vi "#SPI_TOF_LIDAR_cz_test.vi"() -> ()   [LabVIEW 2020]
uses:
  <vilib>/Analysis/baseanly.llb/Mean (DBL).vi
  handle_ALP_error.vi
  <vilib>/Utility/error.llb/Error Cluster From Error Code.vi
  <vilib>/Analysis/NI_AALBase.lvlib
  <vilib>/gmath/NI_Gmath.lvlib
panel:
  out "Trigger Delay (samples)":u32
  out "Rapid Block Acquisition Settings":T1={"preTriggerSamples"=0, "postTriggerSamples"=1000, "timebase"=2, "Four Channel Device"=FALSE, "Oversample"=1, "Number of Captures"=1}
  in  "Tab Control 2":T2(tab)
  out "Resolution":i32=32 min=16 max=128 step=16
  in  "Max Resolution":enum16{"128", "64", "32", "16"}(ring)=enum."32"
  in  "Pulses/Pattern":i32=4
  in  "Trigger Settings":T3={"Trigger Enabled"=TRUE, "Trigger Source"=enum."Channel C", "Trigger Threshold"=10, "Trigger Direction"=2, "Trigger Delay (samples)"=40, "Auto Trigger Time (ms)"=1000} {"Trigger Direction" items=["Rising"=2, "Falling"=3]}
  out "Captures":u32=10240
  in  "Post Trig. Samples":u32=30
  out "Patterns Loaded":dbl(slide)=2048.0 scale=0.0..2048.0
  in  "Initialised?":bool
  in  "y":dbl=0.9
  out "picture time s":dbl=0.0005142857142857143 format="%#.3p"
  in  "Pre Trigger Samples":u32
  in  "Patterns":enum16{"Hadamard", "Random", "Democratised"}(ring)
  in  "Smooth (pixels)":dbl=0.4 format="%#_13g"
  in  "ntimes":i32=4
  in  "Thresholded":bool
  in  "First":bool
  in  "upsample factor":i32=1
  in  "Depth Smooth":dbl=1.0 format="%#_13g"
  in  "depth threshold":dbl=1.0000000000000009
  in  "reflectivity threshold":dbl=0.35 format="%#_13g"
  in  "max reflectivity":dbl=1.0
  in  "index (row)":i32
  in  "Additional Data":dbl=1.25 format="%#_13g"
  out "# elements 2":i32
  out "Total Rate (Hz)":dbl=45.45454545454545 format="%.2g"
  out "# elements 3":i32
  out "2D Rate (Hz)":dbl=inf format="%.2g"
  out "3D Rate (Hz)":dbl=inf format="%.2g"
  out "Update Rate (Hz)":dbl=45.45454545454545 format="%.2g"
  in  "Tab Control":T4(tab)=enum."Temporal Signals"
  out "?":dbl[](graph)
  out "?":dbl[](graph)
  out "pattern temporal signal":cluster{dbl[], dbl[]}(graph)
  out "?":dbl[](graph)
  out "Depth Map":dbl[][](graph)
  out "Reconstruction":dbl[][](graph)
  out "Hadamards":bool[][](array[boolean])
  in  "Channel A Settings":T5={"Enabled"=TRUE, "Coupling"=2, "Range"=3, "Analogue Offset"=0.0, "Bandwidth"=0} {"Bandwidth" items=["Full", "20 MHz"]; "Range" items=["10 mV", "20 mV", "50 mV", "100 mV", "200 mV", "500 mV", "1 V", "2 V", "5 V", "10 V", "20 V", "50 V ", "100 V"]; "Coupling" items=["AC", "DC 1 MOhm", "DC 50 Ohm"]}
  out "total patterns":i32=2048
  in  "Stop":bool=TRUE
  # "3000"
  # "maxADC=32512"
  # "400ps per delay point"
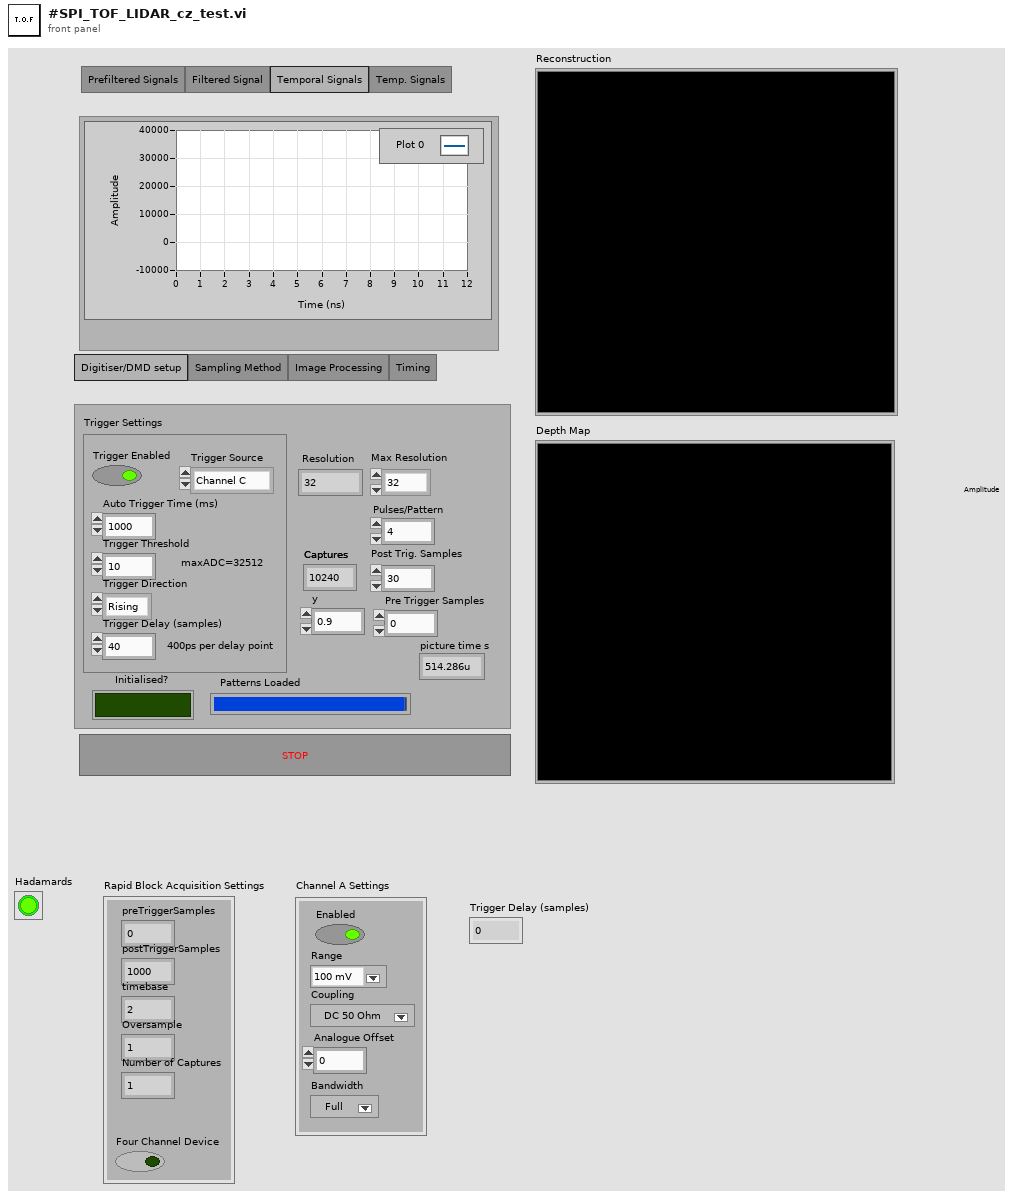
[diagram p1: front panel]
types:
  T1 = cluster{"preTriggerSamples":u32, "postTriggerSamples":u32, "timebase":u32, "Four Channel Device":bool, "Oversample":i16, "Number of Captures":u32}
  T2 = enum32{"Digitiser/DMD setup", "Sampling Method", "Image Processing", "Timing"}
  T3 = cluster{"Trigger Enabled":bool, "Trigger Source":enum32{"Channel A", "Channel B", "Channel C", "Channel D", "External", "Aux."}, "Trigger Threshold":i16, "Trigger Direction":u16, "Trigger Delay (samples)":u32, "Auto Trigger Time (ms)":i16}
  T4 = enum32{"Prefiltered Signals", "Filtered Signal", "Temporal Signals", "Temp. Signals"}
  T5 = cluster{"Enabled":bool, "Coupling":u32, "Range":u32, "Analogue Offset":sgl, "Bandwidth":u32}
  T6 = cluster{dbl[][], "All Patterns out":bool[][], "LUT":i32[]}
  T7 = typedef "imagedata.ctl" = cluster{"image type":i32, "image depth":i32, "image":u8[], "mask":u8[], "colors":u32[], "Rectangle":cluster{"left":i16, "top":i16, "right":i16, "bottom":i16}}
  T8 = cluster{"Pre Trigger Samples":u32, "Post Trig. Samples":u32, "timebase":u32, "Four Channel Device":bool, "Oversample":i16, u32}
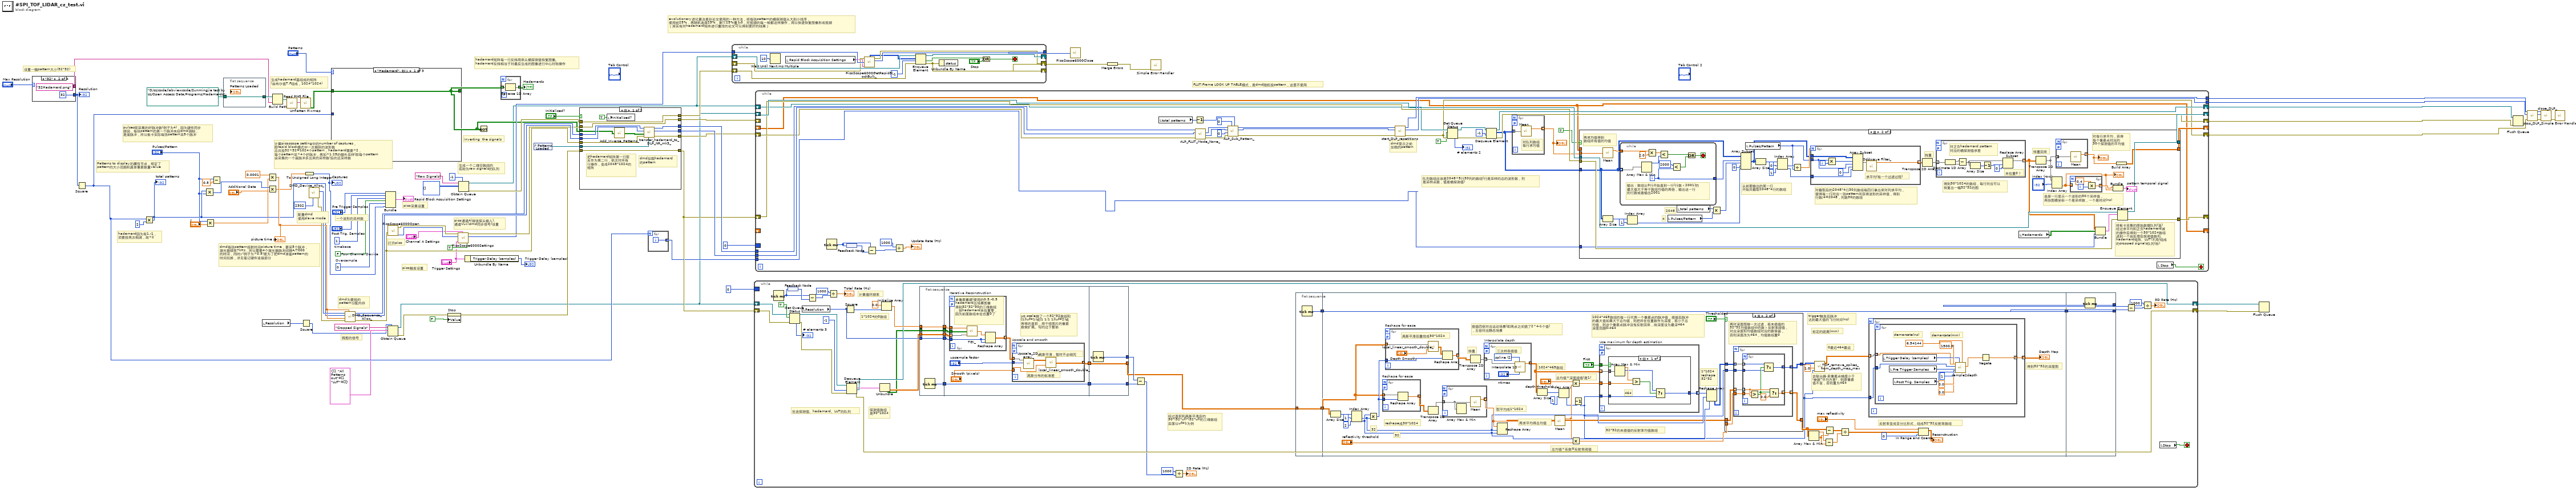
[diagram p0: block diagram]
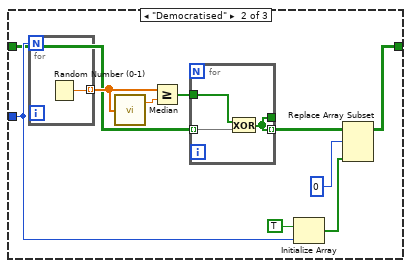
[diagram p2: hidden frame]
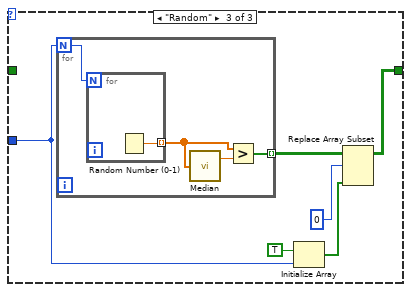
[diagram p3: hidden frame]
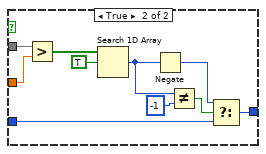
[diagram p5: hidden frame]
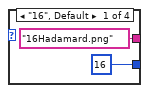
[diagram p8: hidden frame]
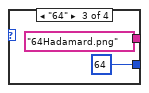
[diagram p9: hidden frame]
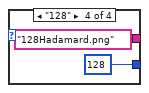
[diagram p10: hidden frame]
diagram:
  w10 = FALSE  # Four Channel Device
  w11 = u32 1  # timebase
  w8 = i16 0  # Oversample
  # "hadamard矩阵每一行反转用来从桶探测值恢复图像。\nhadamard反转相当于对最后生成的图像进行中心对称操作"
  # "pulses即采集的好脉冲数(例子为4)，因为硬件同步\n原因，每张pattern的第一个脉冲未经dmd调制，\n是废脉冲，所以板卡实际每张pattern采5个脉冲"
  # "裁剪的信号"
  # "evolutionary进化算法是孙论文使用的一种方法，将每张pattern的桶探测值从大到小排序，\n使用前25%，再随机选择25%，剩下25%置为0，对视频的每一帧都这样操作，用以快速恢复图像形成视频\n（其实有对hadamard矩阵进行重排的论文可以得到更好的结果）"
  # "生成一个二维空数组的\n名称为raw signals的队列"
  # "FLUT:Frame LOOK UP TABLE模式，是dmd随机投pattern，这里不使用"
  # "pico采集设置"
  # "pico通道A(接收探头输入).\n通道Vux(dmd同步信号)设置"
  # "pico触发设置"
  # "打开pico"
  # "配置dmd\n使用slave mode"
  # "dmd为要投的\npattern分配内存"
  # "dmd每张pattern投射时间picture time，要采5个脉冲，\n激光器频率7kHz，所以需要4个激光器脉冲间隔4/7000\n的时间，同时y(例子为×0.9)是为了把dmd准备pattern的\n时间扣掉，详见笔记硬件连接部分"
  # "一个波形的采样数"
  # "计算picoscope setting中的number of captures，\n即rapid block模式中一次捕获的波形数\n总共投32×32=1024个pattern，hadamard需要×2，\n每个pattern采×4个好脉冲，再加×1.25的额外采样(即每个pattern\n会采集的一个废脉冲多出来的采样数)后的总采样数"
  # "hadamard因为有1.-1，\n须要投两次相减，故×2"
  # "Patterns to display的属性节点，规定了\npattern的大小范围和具体像素数量value"
  # "生成hadamard基组成的矩阵\n(由布尔值T.F组成，1024*1024)"
  # "设置一幅pattern大小(32*32)"
  # "inverting  the signals"
  n1 = case shown="\"32\"" "Max Resolution" {
    tunnel: [16 32 64 128] -> w36
    tunnel: ["16Hadamard.png" ("string") "32Hadamard.png" ("string") "64Hadamard.png" ("string") "128Hadamard.png" ("string")] -> w24
    frame "16", Default {
    }
    frame "32" {
    }
    frame "64" {
    }
    frame "128" {
    }
  }
  "Resolution" <- w36
  n2 = Square(x=w36) -> (x^2=w34:i32)
  n3 = Multiply(x=w34, y=2) -> (x*y=w35:i32)
  "total patterns" <- w35
  n4 = Multiply(x=w35, y="Pulses/Pattern") -> (x*y=w54:i32)
  n5 = Multiply(x="Pulses/Pattern", y="y") -> (x*y=w20:dbl)
  n6 = Subtract(x="Pulses/Pattern", y=0.5) -> ()  [unwired: 1 out]
  n7 = flat-sequence {
    tunnel: path "D:/cz/code/labviewcode/Sunmingjie test by cz/Open Access Data/Programs/Hadamards" ("Folder to Store Files 2") -> [w91]
    tunnel: [w91] -> w25
    frame #0 {
    }
  }
  n8 = local read "Resolution"() -> (w52:i32)
  n9 = Multiply(x=0.0001, y=w20) -> (x*y=w76:dbl)
  "picture time s" <- w76
  n10 = Multiply(x=w54, y="Additional Data") -> (x*y=w60:dbl)
  n11 = Build Path(base path=w25, name or relative path=w24) -> (appended path=w23:path)
  n12 = call <vilib>:"Read PNG File.vi"("path to PNG file"=w23) -> ("image data"=w27:T7)  [unwired: 8 in, 2 out]
  n13 = call <vilib>:"Unflatten Pixmap.vi"("image data"=w27) -> ("1-bit pixmap"=w26:bool[][])  [unwired: 4 in, 6 out]
  n14 = Square(x=w52) -> (x^2=w16:i32)
  n15 = To Unsigned Long Integer(number=w60) -> (unsigned 32bit integer=w7:u32)
  "Captures" <- w7
  n16 = call "DMD_Device_Alloc_.vi"("Master/Slave Mode"=2302) -> ("error out"=w81:errorcluster, "DeviceIdPtr"=w82:u32)  [unwired: 8 in, 1 out]
  n17 = case shown="\"Hadamard\", 默认" "Patterns" {
    tunnel: w34 -> [_ w102 w108]
    tunnel: [w92 w98 w107] -> w18
    tunnel: w26 -> [w92 w96 _]
    frame "Hadamard", Default {
    }
    frame "Democratised" {
      n18 = for {
        N: w102 -> [_]
        tunnel: [w106] -> w97 mode=indexing
        n19 = Random Number (0-1)() -> (number: 0 to 1=w106:dbl)
      }
      n20 = call <vilib>:"Median.vi"("X"=w97) -> ("median"=w94:dbl)  [unwired: 1 out]
      n21 = Greater Or Equal?(x=w97, y=w94) -> (x >= y?=w93:bool[])
      n22 = for {
        tunnel: w93 -> [w105]
        tunnel: w96 -> [w104] mode=indexing
        tunnel: [w103] -> w95 mode=indexing
        tunnel: [w103] -> _
        n23 = Exclusive Or(1:w104, 2:w105) -> (0:w103:bool[])
      }
      n24 = Initialize Array(TRUE, w102) -> (w100:bool[])
      n25 = Replace Array Subset(array=w95, new element=w100, index (row)=0) -> (w98:bool[][])  [unwired: 1 in]
    }
    frame "Random" {
      n26 = for {
        N: w108 -> [w116]
        tunnel: [w113] -> w110 mode=indexing
        n27 = for {
          N: w116 -> [_]
          tunnel: [w117] -> w114 mode=indexing
          n28 = Random Number (0-1)() -> (number: 0 to 1=w117:dbl)
        }
        n29 = call <vilib>:"Median.vi"("X"=w114) -> ("median"=w115:dbl)  [unwired: 1 out]
        n30 = Greater?(x=w114, y=w115) -> (0:w113:bool[])
      }
      n31 = Initialize Array(TRUE, w108) -> (w111:bool[])
      n32 = Replace Array Subset(array=w110, new element=w111, index (row)=0) -> (w107:bool[][])  [unwired: 1 in]
    }
  }
  n33 = call "DMD_Sequence_Alloc_.vi"("Picture Time (s)"=w76, "error in (no error)"=w81, "Illuminate Time (s)"=w76, "Number of Frames"=w35, "DeviceIdPtr in"=w82) -> ("error out"=w38:errorcluster, "SequenceId"=w73:u32, "DeviceIdPtr out"=w74:u32)  [unwired: 3 in, 1 out]
  n34 = Bundle("Pre Trigger Samples"="Pre Trigger Samples", "Post Trig. Samples"="Post Trig. Samples", "timebase"=w11, "Four Channel Device"=w10, "Oversample"=w8, w7) -> (→"Rapid Block Acquisition Settings":T8)  [unwired: 1 in]
  n35 = call "PicoScope6000Open.vi"("error in (no error)"=w38) -> ("handle"=w62:i16, "error out"=w63:errorcluster)  [unwired: 2 in, 2 out]
  n36 = Obtain Queue(max queue size (-1, unlimited)=w16, name (unnamed)="Cropped Signals", element data type=T6 {[], "All Patterns out"=[], "LUT"=[]} ("output cluster")) -> (queue out=w14:refnum<queue>, error out=w41:errorcluster)  [unwired: 2 in, 1 out]
  n37 = property on="Stop" class="Bool (严格)"(error in=w41, "Value"=FALSE ("Stop")) -> (error out=w40:errorcluster)  [unwired: 1 in, 1 out]
  n38 = call "PicoScope6000Settings.vi"("PS6407?"=TRUE, "Channel A Settings"="Channel A Settings", "Trigger Settings"="Trigger Settings", "handle in"=w62, "error in"=w63) -> ("handle out"=w45:i16, "error out"=w48:errorcluster)  [unwired: 4 in, 1 out]
  n39 = Obtain Queue(max queue size (-1, unlimited)=-1, name (unnamed)="Raw Signals", element data type=i16[][] [] ("Channel A Buffer")) -> (queue out=w15:refnum<queue>, error out=w47:errorcluster)  [unwired: 2 in, 1 out]
  n40 = Unbundle By Name("Trigger Settings") -> ("Trigger Delay (samples)"=→"Trigger Delay (samples)":u32)
  n41 = Not(x=w18) -> ()  [unwired: 1 out]
  n42 = for {
    tunnel: w18 -> [w119] mode=indexing
    tunnel: [w118] -> w17 mode=indexing
    n43 = Reverse 1D Array(array=w119) -> (reversed array=w118:bool[])
  }
  "Hadamards" <- w17
  n44 = control-ref of="Patterns Loaded"() -> (w69:refnum<vi>)
  n45 = case shown="假" "Initialised?" {
    tunnel: w74 -> [w131 w138]
    tunnel: w38 -> [w130 w137]
    tunnel: [w127 w138] -> w72
    tunnel: [w126 w136] -> w71
    tunnel: [w128 w137] -> w55
    tunnel: w69 -> [w129 _]
    tunnel: w73 -> [w125 w136]
    tunnel: w18 -> [w124 _]
    tunnel: [w122 w135] -> w44
    tunnel: w48 -> [w122 w135]
    tunnel: [w121 w134] -> w46
    tunnel: w47 -> [w121 w134]
    tunnel: w40 -> [w120 w133]
    tunnel: [w120 w133] -> w39
    frame False {
      # "dmd加载hadamard\n的pattern"
      # "把hadamard矩阵第一行取\n反作为第二行，依次对所有\n行操作，变成2048*1024的\n矩阵"
      n46 = local write "Initialised?"(TRUE ("Initialised?")) -> ()
      n47 = call "Add_Inverse_Patterns_.vi"("Hadamard"=w124) -> ("Array"=w123:bool[][])
      n48 = call "transfer_hadamard_to_DLP_NR_mk3_.vi"("Progress Indicator"=w129, "error in (no error)"=w130, "Hadamard"=w123, "SequenceId"=w125, "DeviceId"=w131) -> ("error out"=w128:errorcluster, "SequenceId Out"=w126:u32, "DeviceId Out"=w127:u32)  [unwired: 4 in]
    }
    frame True {
    }
  }
  n49 = for {
    N: w34 -> [_]
    tunnel: [w139] -> w37 mode=indexing
    i -> [w139]
  }
  n50 = while {
    shift-right: [w152] -> _
    shift-left: w15 -> [w153]
    tunnel: w45 -> [w151]
    shift-right: [w147] -> _
    shift-left: _ -> [w146]
    shift-right: [w145] -> w57
    shift-left: w46 -> [w148]
    tunnel: [w143] -> w56
    stop <- w144 stop-if-true
    n51 = Wait Until Next ms Multiple(millisecond multiple=u32 10) -> ()  [unwired: 1 out]
    n52 = local read "Rapid Block Acquisition Settings"() -> (w140:T1)
    n53 = call "PicoScope6000GetRapidBlockBulk_.vi"("error in"=w146, "handle in"=w151, "Rapid Block Acquisition Settings"=w140) -> ("Channel A Buffer"=w142:i16[][], "error out"=w147:errorcluster, "handle out"=w143:i16)  [unwired: 7 in, 3 out]
    n54 = Enqueue Element(queue=w153, element=w142, timeout in ms (-1)=-1, error in (no error)=w148) -> (queue out=w152:refnum<queue>, timed out?=w149:bool, error out=w145:errorcluster)
    n55 = Unbundle By Name(w145) -> ()  [unwired: 1 out]
    n56 = Or(x=w149, y="Stop") -> (x .or. y?=w144:bool)
  }
  n57 = while {
    shift-right: [w191] -> w31
    shift-left: w14 -> [w182]
    shift-right: [w189] -> w30
    shift-left: w39 -> [w181]
    border: u32 0 ("millisecond timer value") -> [_]
    stop <- w193 stop-if-true
    # "经过直积和高斯平滑后的\n30*(32*uf)*(32*uf)的三维数组\n后面以uf=1为例"
    # "探测值数组\n是30*1024"
    # "包含探测值、hadamard、LUT的队列"
    # "1*1024的0数组"
    # "计算循环频率"
    n58 = Tick Count (ms)() -> (millisecond timer value=w187:u32)
    n59 = feedback #1() -> (w188:u32)
    n60 = feedback-in #1(w187) -> ()
    n61 = Get Queue Status(queue=w182, return elements? (F)=TRUE, error in (no error)=w181) -> (queue out=w180:refnum<queue>, error out=w179:errorcluster, # elements in queue=→"# elements 3":i32)  [unwired: 5 out]
    n62 = local read "Resolution"() -> (w192:i32)
    n63 = Subtract(x=w187, y=w188) -> (x-y=w186:u32)
    n64 = Divide(x=u32 1000, y=w186) -> (x/y=→"Total Rate (Hz)":dbl)
    n65 = Square(x=w192) -> (x^2=w197:i32)
    n66 = Dequeue Element(queue=w180, timeout in ms (-1)=-1, error in (no error)=w179) -> (queue out=w191:refnum<queue>, element=w190:T6, error out=w189:errorcluster)  [unwired: 1 out]
    n67 = Unbundle(w190) -> (w156:dbl[][], "All Patterns out"=w155:bool[][])  [unwired: 1 out]
    n68 = Initialize Array(0.0 ("element"), w197) -> (w195:dbl[])
    n69 = flat-sequence {
      tunnel: w155 -> [w317]
      tunnel: w156 -> [w318]
      tunnel: w192 -> [w319]
      tunnel: w195 -> [w320]
      tunnel: [w320] -> w177
      tunnel: [w319] -> w176
      tunnel: [w318] -> w175
      tunnel: [w317] -> w174
      tunnel: [w316] -> w167
      tunnel: w177 -> [w329]
      tunnel: w176 -> [w328]
      tunnel: w175 -> [w326]
      tunnel: w174 -> [w325]
      tunnel: [w322] -> w173
      tunnel: w167 -> [w321]
      tunnel: [w321] -> w166
      tunnel: [w343] -> w165
      tunnel: w173 -> [w343]
      tunnel: [w342] -> w169
      tunnel: [w341] -> w168
      tunnel: w166 -> [w341]
      frame #0 {
        n70 = Tick Count (ms)() -> (millisecond timer value=w316:u32)
      }
      frame #1 {
        # "up scale做了一个32*32数组和\n[1](uf=1)或[1 1;1 1](uf=2)或\n等等的直积，用于将图片的像素\n数做扩展。写的过于繁琐"
        n71 = for "Iterative Reconstruction" {
          tunnel: w326 -> [w336] mode=indexing
          tunnel: w328 -> [w340]
          tunnel: [w338] -> w324 mode=indexing
          tunnel: w329 -> [w339]
          tunnel: w325 -> [w337]
          workers-P: _ -> [_]
          # "单像素重建(使用的0.5,-0.5\nhadamard出场景图像\n得到32*32*30的三维数组\n，但hadamard末位置零，\n因为前面数组末位也置0了"
          n72 = call "TGI_.vi"("Signals"=w336, "Hadamard"=w337, "Initialise Array"=w339) -> ("Reconstruction"=w335:dbl[])
          n73 = Reshape Array(w335, w340, w340) -> (w338:dbl[][])
        }
        n74 = for "Upscale and smooth" {
          tunnel: w324 -> [w334] mode=indexing
          tunnel: "Smooth (pixels)" -> [w333]
          tunnel: [w331] -> w322 mode=indexing
          tunnel: "upsample factor" -> [w330]
          workers-P: _ -> [_]
          # "高斯分布的标准差"
          # "高斯平滑，暂时不必细究"
          n75 = call "Upscale_2D_array_.vi"("Upsample Factor"=w330, "Small Array"=w334) -> ("Big Array"=w332:dbl[][])  [unwired: 7 in, 2 out]
          n76 = call "local_linear_smooth_double_.vi"("Smoothing Parameter (Gaussian S.D. in pixels)"=w333, "Input Array"=w332) -> ("Smoothed Array"=w331:dbl[][])
        }
      }
      frame #2 {
        n77 = Tick Count (ms)() -> (millisecond timer value=w342:u32)
      }
    }
    n78 = Subtract(x=w169, y=w168) -> (x-y=w170:u32)
    n79 = Divide(x=u32 1000, y=w170) -> (x/y=→"2D Rate (Hz)":dbl)
    n80 = flat-sequence {
      tunnel: w165 -> [w199]
      tunnel: [w199] -> w164
      tunnel: [w198] -> w159
      tunnel: w164 -> [w207]
      tunnel: [w223] -> w160
      tunnel: w159 -> [w223]
      tunnel: [w315] -> w158
      tunnel: w160 -> [w315]
      tunnel: [w314] -> w157
      frame #0 {
        n81 = Tick Count (ms)() -> (millisecond timer value=w198:u32)
      }
      frame #1 {
        # "标定的距离(mm)"
        # "trigger触发后脉冲\n达到最大值的飞行时间(ns)"
        # "0最近464最远"
        # "得到32*32的深度图"
        # "去除尖峰,若像素点梯度小于\n(参数*平均方差)，则原像素\n值不变，否则置为464"
        # "反射率变成百分比形式，组成32*32反射率数组"
        # "1*1024\nreshape\n32*32"
        # "32"
        # "32"
        # "reshape成30*1024"
        # "1024*465数组的每一行代表一个像素点的脉冲值，插值后脉冲\n的最大值如果大于总均值，则把所在位置数作为深度，若小于总\n均值，则这个像素点脉冲没有反射回来，故深度设为最深464\n深度范围0-464"
        # "1024*465数组"
        # "转置"
        # "32*32的未插值的反射率均值数组"
        # "总均值×深度阈值(是1)"
        # "总均值×系数=反射率阈值"
        # "再求平均得总均值"
        # "取平均成1*1024"
        # "插值四倍对应运动场景(即两点之间插了2^4-1个值)\n，五倍对应静态场景"
        n82 = Array Size(array=w207) -> (size(s)=w240:i32[])
        n83 = Index Array(array=w240, index #1=1 ("index"), index #2=2 ("index")) -> (element #1=w234:i32, element #2=w233:i32)
        n84 = Multiply(x=w233, y=w234) -> (x*y=w227:i32)
        n85 = for "Reshape for ease" {
          tunnel: w207 -> [w309] mode=indexing
          tunnel: w227 -> [w308]
          tunnel: [w307] -> w237 mode=indexing
          workers-P: _ -> [_]
          n86 = Reshape Array(w309, w308) -> (w307:dbl[])
        }
        n87 = for "Reshape for ease" {
          tunnel: w227 -> [w256]
          tunnel: [w260] -> w225 mode=indexing
          tunnel: w207 -> [w259] mode=indexing
          workers-P: _ -> [_]
          # "高斯平滑后重排成30*1024"
          n88 = call "local_linear_smooth_double_.vi"("Smoothing Parameter (Gaussian S.D. in pixels)"="Depth Smooth", "Input Array"=w259) -> ("Smoothed Array"=w258:dbl[][])
          n89 = Reshape Array(w258, w256) -> (w260:dbl[])
        }
        n90 = Transpose 2D Array(2D array=w237) -> (transposed array=w236:dbl[][])
        n91 = for {
          tunnel: w236 -> [w284] mode=indexing
          tunnel: [w283] -> w235 mode=indexing
          workers-P: _ -> [_]
          n92 = Array Max & Min(array=w284) -> ()  [unwired: 4 out]
          n93 = call-poly <vilib>:"Mean.vi"("X"=w284) -> ("mean"=w283:dbl)  [unwired: 1 out]
        }
        n94 = Transpose 2D Array(2D array=w225) -> (transposed array=w226:dbl[][])
        n95 = for "Interpolate depth" {
          tunnel: w226 -> [w313] mode=indexing
          tunnel: [w311] -> w222 mode=indexing
          workers-P: _ -> [_]
          w312 = 2 items=["nearest", "linear", "spline", "cubic Hermite", "Lagrange"] ("method")
          # "三次样条插值"
          n96 = call <vilib>:"Interpolate 1D.vi"("ntimes"="ntimes", "method"=w312, "Y"=w313) -> ("yi"=w311:dbl[])  [unwired: 6 in, 2 out]
        }
        n97 = Reshape Array(w235, w234, w233) -> (w231:dbl[][])
        n98 = Array Size(array=w222) -> (size(s)=w221:i32[])
        n99 = call-poly <vilib>:"Mean.vi"("X"=w235) -> ("mean"=w218:dbl)  [unwired: 1 out]
        n100 = Index Array(array=w221, index=1) -> (element=w202:i32)
        n101 = Multiply(x="depth threshold", y=w218) -> (x*y=w229:dbl)
        n102 = Multiply(x=w218, y="reflectivity threshold") -> (x*y=w216:dbl)
        n103 = Decrement(x=w202) -> (x-1=w201:i32)
        n104 = for "Use maximum for depth estimation" {
          tunnel: w222 -> [w286] mode=indexing
          tunnel: [w288] -> w224 mode=indexing
          tunnel: w229 -> [w289]
          workers-P: _ -> [_]
          tunnel: w201 -> [w287]
          tunnel: "First" -> [w285]
          n105 = case shown="假" w285 {
            tunnel: w289 -> [w294 w306]
            tunnel: [w291 w300] -> w288
            tunnel: w287 -> [w292 w298]
            tunnel: w286 -> [w296 w297]
            frame False {
              # "464"
              n106 = Array Max & Min(array=w296) -> (max value=w295:dbl, max index (indices)=w290:i32)  [unwired: 2 out]
              n107 = Greater?(x=w295, y=w294) -> (0:w293:bool)
              n108 = Select(t=w290, s=w293, f=w292) -> (s? t:f=w291:i32)
            }
            frame True {
              n109 = Greater?(x=w297, y=w306) -> (0:w305:bool[])
              n110 = Search 1D Array(1D array=w305, element=TRUE) -> (index of element=w299:i32)  [unwired: 1 in]
              n111 = Negate(x=w299) -> (-x=w301:i32)
              n112 = Not Equal?(x=w299, y=-1) -> (x != y?=w302:bool)
              n113 = Select(t=w301, s=w302, f=w298) -> (s? t:f=w300:i32)
            }
          }
        }
        n114 = Reshape Array(w224, w234, w233) -> (w230:i32[][])
        n115 = case shown="真" "Thresholded" {
          tunnel: w231 -> [w262 w267]
          tunnel: w216 -> [_ w268]
          tunnel: [w262 w263] -> w211
          tunnel: w230 -> [w261 w266]
          tunnel: [w261 w264] -> w203
          tunnel: w201 -> [_ w265]
          frame False {
          }
          frame True {
            # "再对深度图做一次过滤，若未插值的\n32*32均值数组中的数＞反射率阈值，\n对应深度和均值数组对应的数保留，\n否则深度改为464，均值数组置0"
            n116 = for {
              tunnel: [w274] -> w263 mode=indexing
              tunnel: w267 -> [w273] mode=indexing
              tunnel: w268 -> [w272]
              tunnel: w266 -> [w271] mode=indexing
              tunnel: w265 -> [w269]
              tunnel: [w270] -> w264 mode=indexing
              n117 = for {
                tunnel: [w282] -> w274 mode=indexing
                tunnel: w273 -> [w280] mode=indexing
                tunnel: w272 -> [w281]
                tunnel: w271 -> [w277] mode=indexing
                tunnel: w269 -> [w276]
                tunnel: [w275] -> w270 mode=indexing
                n118 = Greater?(x=w280, y=w281) -> (0:w278:bool)
                n119 = Select(t=w277, s=w278, f=w276) -> (s? t:f=w275:i32)
                n120 = Select(t=w280, s=w278, f=0.0) -> (s? t:f=w282:dbl)
              }
            }
          }
        }
        n121 = Array Max & Min(array=w211) -> (max value=w215:dbl, min value=w214:dbl)  [unwired: 2 out]
        n122 = call "TOF_remove_spikes_from_depth_map_max.vi"("max"=w201, "threshold for spike removal (standard deviations)"=1.0, "Depth Map"=w203) -> ("Depth Map (no spikes)"=w206:dbl[][])  [unwired: 8 in]
        n123 = Subtract(x=w215, y=w214) -> (x-y=w212:dbl)
        n124 = Subtract(x=w211, y=w214) -> (x-y=w213:dbl[][])
        n125 = Divide(x=w213, y=w212) -> (x/y=w210:dbl[][])
        n126 = for {
          tunnel: w206 -> [w243] mode=indexing
          tunnel: w201 -> [w242]
          tunnel: [w241] -> w200 mode=indexing
          n127 = for {
            tunnel: w243 -> [w252] mode=indexing
            tunnel: w242 -> [w251]
            tunnel: [w244] -> w241 mode=indexing
            # "demarcate(mm)"
            # "demarcate(ns)"
            n128 = local read "Trigger Delay (samples)"() -> (w253:u32)
            n129 = local read "Pre Trigger Samples"() -> (w250:u32)
            n130 = local read "Post Trig. Samples"() -> (w249:u32)
            n131 = call "sample2depth.vi"("min"=0.0, "demarcate(mm)"=1500.0, "correct(mm)"=0.0, "demarcate(ns)"=6.54144 ("demarcate(sample)"), "timebase(0-4)"=u32 1, "Trigger Delay (samples)"=w253, "Post Trig. Samples"=w249, "Pre Trigger Samples"=w250, "max"=w251, "sample"=w252) -> ("depth"=w245:dbl)  [unwired: 1 in]
            n132 = Negate(x=w245) -> (-x=w244:dbl)
          }
        }
        "Depth Map" <- w200
        n133 = In Range and Coerce(upper limit="max reflectivity", x=w210, lower limit=0 ("index (row)")) -> (coerced(x)=→"Reconstruction":dbl[][])  [unwired: 1 out]
      }
      frame #2 {
        n134 = Tick Count (ms)() -> (millisecond timer value=w314:u32)
      }
    }
    n135 = Subtract(x=w157, y=w158) -> (x-y=w161:u32)
    n136 = Divide(x=u32 1000, y=w161) -> (x/y=→"3D Rate (Hz)":dbl)
    n137 = local read "Stop"() -> (w193:bool)
  }
  n138 = while {
    tunnel: w72 -> [w383]
    tunnel: w71 -> [w380]
    tunnel: [w382] -> w68
    tunnel: [w381] -> w67
    tunnel: w37 -> [w370]
    shift-right: [w378] -> w51
    shift-left: w15 -> [w368]
    shift-right: [w367] -> w50
    shift-left: w55 -> [w377]
    shift-right: [w375] -> _
    shift-left: w14 -> [w374]
    shift-right: [w373] -> _
    shift-left: w39 -> [w372]
    shift-right: [w369] -> _
    shift-left: _ -> [w362]
    shift-right: [w371] -> w43
    shift-left: w44 -> [_]
    shift-right: [w362] -> _
    shift-left: _ -> [_]
    border: u32 0 ("millisecond timer value") -> [_]
    stop <- w379 stop-if-true
    # "dmd显示之前\n加载的pattern"
    # "队列数组应该是2048×5行30列的数组(行是采样的总的波形数，列\n是采样点数，值是桶探测值)"
    n139 = Tick Count (ms)() -> (millisecond timer value=w347:u32)
    n140 = feedback #2() -> (w348:u32)
    n141 = feedback-in #2(w347) -> ()
    n142 = Subtract(x=w347, y=w348) -> (x-y=w346:u32)
    n143 = Divide(x=u32 1000, y=w346) -> (x/y=→"Update Rate (Hz)":dbl)
    n144 = local read "total patterns"() -> (w353:i32)
    n145 = Decrement(x=w353) -> (x-1=w352:i32)
    n146 = call "ALP_FLUT_Mode_None_.vi"("error in (no error)"=w377, "SequenceId in"=w380, "DeviceId in"=w383) -> ("error out"=w351:errorcluster, "SequenceId out"=w350:u32, "DeviceId out"=w349:u32)  [unwired: 6 in]
    n147 = call "ALP_Sub_Pattern_.vi"("Last Frame"=w352, "First Frame"=0, "error in (no error)"=w351, "Repetitions"=0, "SequenceId in"=w350, "DeviceIdPtr in"=w349) -> ("error out"=w357:errorcluster, "SequenceId out"=w354:u32, "DeviceId"=w358:u32)  [unwired: 3 in]
    n148 = call "start_DLP_repetitions.vi"("error in (no error)"=w357, "SequenceId"=w354, "DeviceId"=w358) -> ("error out"=w367:errorcluster, "SequenceId Out"=w381:u32, "DeviceId Out"=w382:u32)  [unwired: 6 in]
    n149 = Get Queue Status(queue=w368, return elements? (F)=TRUE, error in (no error)=w367) -> (queue out=w366:refnum<queue>, error out=w365:errorcluster, # elements in queue=→"# elements 2":i32)  [unwired: 5 out]
    n150 = Dequeue Element(queue=w366, timeout in ms (-1)=-1, error in (no error)=w365) -> (queue out=w378:refnum<queue>, element=w359:i16[][], error out=w371:errorcluster)  [unwired: 1 out]
    n151 = for {
      tunnel: w359 -> [w455] mode=indexing
      tunnel: [w454] -> w360 mode=indexing
      workers-P: _ -> [_]
      # "对队列数组\n每行求均值"
      n152 = call-poly <vilib>:"Mean.vi"("X"=w455) -> ("mean"=w454:dbl)  [unwired: 1 out]
    }
    "?" <- w360
    n153 = case shown="真" TRUE {
      tunnel: [w386 w422] -> w375
      tunnel: w374 -> [w386 w421]
      tunnel: [w385 w420] -> w373
      tunnel: w372 -> [w385 w419]
      tunnel: w370 -> [_ w393]
      tunnel: [w384 w416] -> w369
      tunnel: w360 -> [_ w396]
      tunnel: w359 -> [_ w394]
      tunnel: w362 -> [w384 _]
      frame False {
      }
      frame True {
        # "4"
        # "2048"
        # "转置回来"
        # "将板卡采集的原始数据队列(蓝)\n经过求平均和正负hadamard减\n的操作后得到一个30*1024数组\n送到一个由处理后探测值数列、\nhadamard矩阵、LUT(不用)组成\n的cropped signals队列(粉)"
        # "对每行求平均，获得\n每个像素点对应的\n30个探测值的平均值"
        # "选择一行显示一个波形的30个采样值，\n两张图横坐标一个是采样数，一个是时间(ns)"
        # "转置"
        # "再求均值得到\n数组所有值的均值"
        # "得到30*1024的数组，每行对应可以\n恢复出一幅32*32的图"
        # "从前面输出的某一行\n开始共截取2048*4行的数组"
        # "对截取后的2048*4行30列数组每四行拿出来对列求平均，\n使得每一行对应一张pattern所获得波形的采样值，得到\n行数/4=2048，列数30的数组"
        n154 = call-poly <vilib>:"Mean.vi"("X"=w396) -> ("mean"=w403:dbl)  [unwired: 1 out]
        n155 = Array Size(array=w394) -> (size(s)=w405:i32[])
        n156 = while {
          tunnel: w394 -> [w427] mode=indexing
          tunnel: [w433] -> w388
          tunnel: w403 -> [w426]
          i -> [w433]
          stop <- w429 stop-if-true
          # "输出：数组从0行开始直到一行(行数＜2001)的\n最大值大于等于数组均值的两倍，输出这一行\n的行数或者输出2001"
          n157 = Array Max & Min(array=w427) -> (max value=w428:i16)  [unwired: 3 out]
          n158 = Multiply(x=w426, y=2.0) -> (x*y=w434:dbl)
          n159 = Less?(x=w434, y=w428) -> (x < y?=w430:bool)
          n160 = Less?(x=2000, y=w433) -> (x < y?=w431:bool)
          n161 = Or(x=w430, y=w431) -> (x .or. y?=w429:bool)
        }
        n162 = Index Array(array=w405, index=1) -> (element=w387:i32)
        n163 = local read "Pulses/Pattern"() -> (w401:i32)
        n164 = local read "total patterns"() -> (w402:i32)
        n165 = Multiply(x=w402, y=w401) -> (x*y=w400:i32)
        n166 = Array Subset(array=w394, index (row)=w388, length (row)=w400, index (col)=0 ("index"), length (col)=w387) -> (w406:i16[][])
        n167 = local read "Pulses/Pattern"() -> (w399:i32)
        n168 = Array Size(array=w406) -> (size(s)=w413:i32[])
        n169 = Index Array(array=w413, index #1=0 ("index"), index #2=1 ("index")) -> (element #1=w409:i32, element #2=w408:i32)
        n170 = Divide(x=w409, y=w399) -> (x/y=w410:dbl)
        n171 = for {
          N: w410 -> [_]
          tunnel: w406 -> [w451]
          tunnel: w408 -> [w450]
          tunnel: [w444] -> w397 mode=indexing
          tunnel: w399 -> [w445]
          i -> [w448]
          # "求平均(有一个过滤过程)"
          n172 = Multiply(x=w445, y=w448) -> (x*y=w447:i32)
          n173 = Array Subset(array=w451, index (row)=w447, length (row)=w445, index (col)=0 ("index"), length (col)=w450) -> (w446:i16[][])
          n174 = call "Oddwave Filter_.vi"("Wave Array Input"=w446) -> ("Averaged Wave Output"=w444:dbl[])  [unwired: 8 in, 1 out]
        }
        n175 = Transpose 2D Array(2D array=w397) -> (transposed array=w398:dbl[][])
        n176 = for {
          tunnel: w398 -> [w441] mode=indexing
          tunnel: [w436] -> w395 mode=indexing
          workers-P: _ -> [_]
          # "末位置0？"
          # "对正负hadamard pattern\n对应的桶探测值求差"
          n177 = Decimate 1D Array(w441) -> (w443:dbl[], w442:dbl[])
          n178 = Subtract(x=w443, y=w442) -> (x-y=w437:dbl[])
          n179 = Array Size(array=w437) -> (size(s)=w440:i32)
          n180 = Decrement(x=w440) -> (x-1=w439:i32)
          n181 = Replace Array Subset(array=w437, new element=0 ("new element/subarray"), index=w439) -> (w436:dbl[])
        }
        n182 = local read "Hadamards"() -> (w417:bool[][])
        n183 = Transpose 2D Array(2D array=w395) -> (transposed array=w414:dbl[][])
        n184 = Index Array(array=w414, index (row)="index (row)") -> (element=w389:dbl[])  [unwired: 1 in]
        "?" <- w389
        n185 = for {
          tunnel: w414 -> [w452] mode=indexing
          tunnel: [w453] -> w392 mode=indexing
          workers-P: _ -> [_]
          n186 = call-poly <vilib>:"Mean.vi"("X"=w452) -> ("mean"=w453:dbl)  [unwired: 1 out]
        }
        "?" <- w392
        n187 = for {
          tunnel: [w423] -> w391 mode=indexing
          tunnel: w389 -> [_] mode=indexing
          i -> [w424]
          n188 = Multiply(x=0.4, y=w424) -> (x*y=w423:dbl)
        }
        n189 = Bundle(w395, "Hadamards"=w417, w393) -> (w418:cluster{dbl[][], "Hadamards":bool[][], i32[]})  [unwired: 1 in]
        n190 = Bundle(w391, w389) -> (→"pattern temporal signal":cluster{dbl[], dbl[]})  [unwired: 1 in]
        n191 = Build Array(w392) -> (w416:dbl[][])
        n192 = Enqueue Element(queue=w421, element=w418, error in (no error)=w419) -> (queue out=w422:refnum<queue>, error out=w420:errorcluster)  [unwired: 1 in, 1 out]
      }
    }
    n193 = local read "Stop"() -> (w379:bool)
  }
  n194 = call "PicoScope6000Close.vi"("handle"=w56) -> ()
  n195 = Merge Errors(w57) -> (w58:errorcluster)
  n196 = call <vilib>:"Simple Error Handler.vi"("error in (no error)"=w58) -> ()  [unwired: 4 in, 5 out]
  n197 = Flush Queue(queue=w31, error in (no error)=w30) -> ()  [unwired: 3 out]
  n198 = Flush Queue(queue=w51, error in (no error)=w43) -> ()  [unwired: 3 out]
  n199 = call "stop_DLP_.vi"("error in (no error)"=w50, "SequenceId"=w67, "DeviceId"=w68) -> ("error out"=w66:errorcluster, "SequenceId Out"=w65:u32, "DeviceId Out"=w64:u32)  [unwired: 6 in]
  n200 = call "close_DLP_.vi"("error in (no error)"=w66, "SequenceId"=w65, "DeviceId"=w64) -> ("error out"=w70:errorcluster)  [unwired: 8 in]
  n201 = call <vilib>:"Simple Error Handler.vi"("error in (no error)"=w70) -> ()  [unwired: 4 in, 5 out]
